vi "Y_XZModefying.vi"() -> ()   [LabVIEW 2013]
uses:
  <vilib>/Instr/_visa.llb/VISA Configure Serial Port (Instr).vi
  <vilib>/Native 3D Graph/xcontrol/3DPC_SurfacePlot.xctl
  <vilib>/Analysis/Matrix/NI_Matrix.lvlib
  <vilib>/Analysis/Matrix/Numeric/Conversions/Array To Matrix - RA.vi
panel:
  in  "Path":path
  out "3D Graph":refnum<class "Base Datatype.lvclass">[](xcontrol)
  in  "ZAdjustStep um":dbl format="%#_13g"
  in  "CurrFluctuationTolerance %":dbl format="%#_13g"
  in  "stop":bool
  in  "ZRoughApproachPerStep um":dbl format="%#_13g"
  in  "ZMovThresholdChange %":dbl format="%#_13g"
  in  "ZApproachingThresholdDecline %":dbl format="%#_13g"
  in  "ZApproachPerStep um":dbl format="%#_13g"
  in  "ZAdjustSpeed um/s":dbl format="%#_13g"
  in  "ConstantCurrPIZ":refnum<visa-resource-name>
  in  "ZApproachSpeed um/s":dbl format="%#_13g"
  in  "YMovSpeed um/s":dbl format="%#_13g"
  in  "XMovSpeed um/s":dbl format="%#_13g"
  in  "Y Length / um":dbl format="%#_13g"
  in  "X Length / um":dbl format="%#_13g"
  in  "Y Resolution":i32
  in  "X Resolution":i32
  in  "Amp":refnum<visa-resource-name>
  in  "Moving":refnum<visa-resource-name>
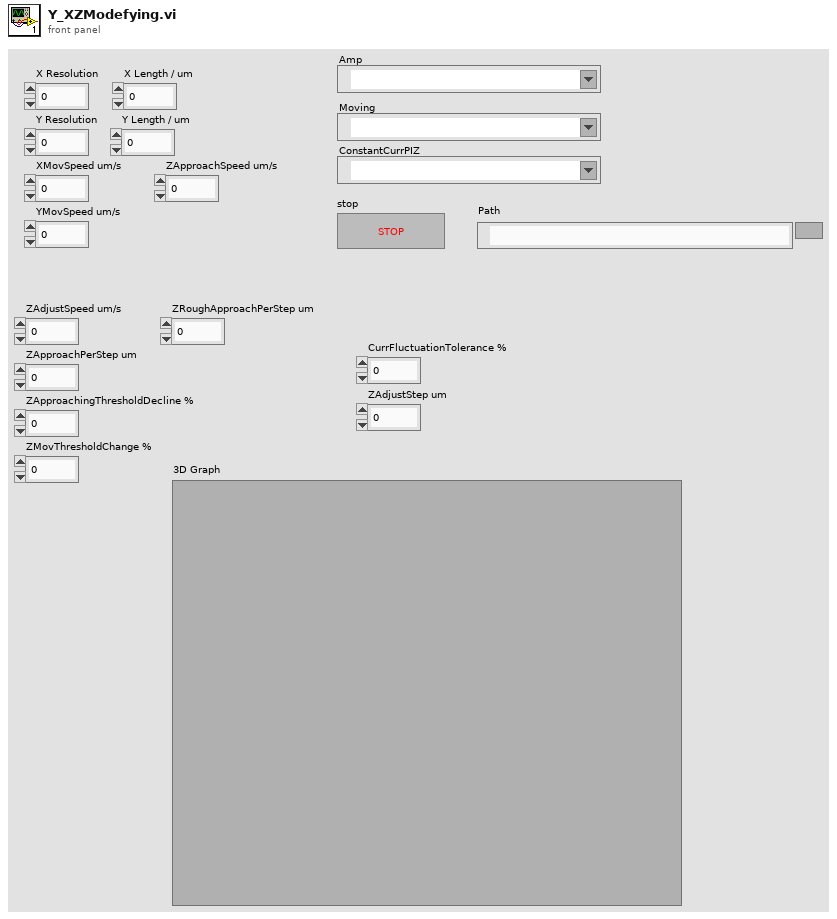
[diagram p1: front panel]
types:
  T1 = enum16{"open", "replace", "create", "open or create", "replace or create", "replace or create with confirmation"}
  T2 = typedef "NI_Matrix.lvlib/RealMatrix.ctl" = dbl[][]
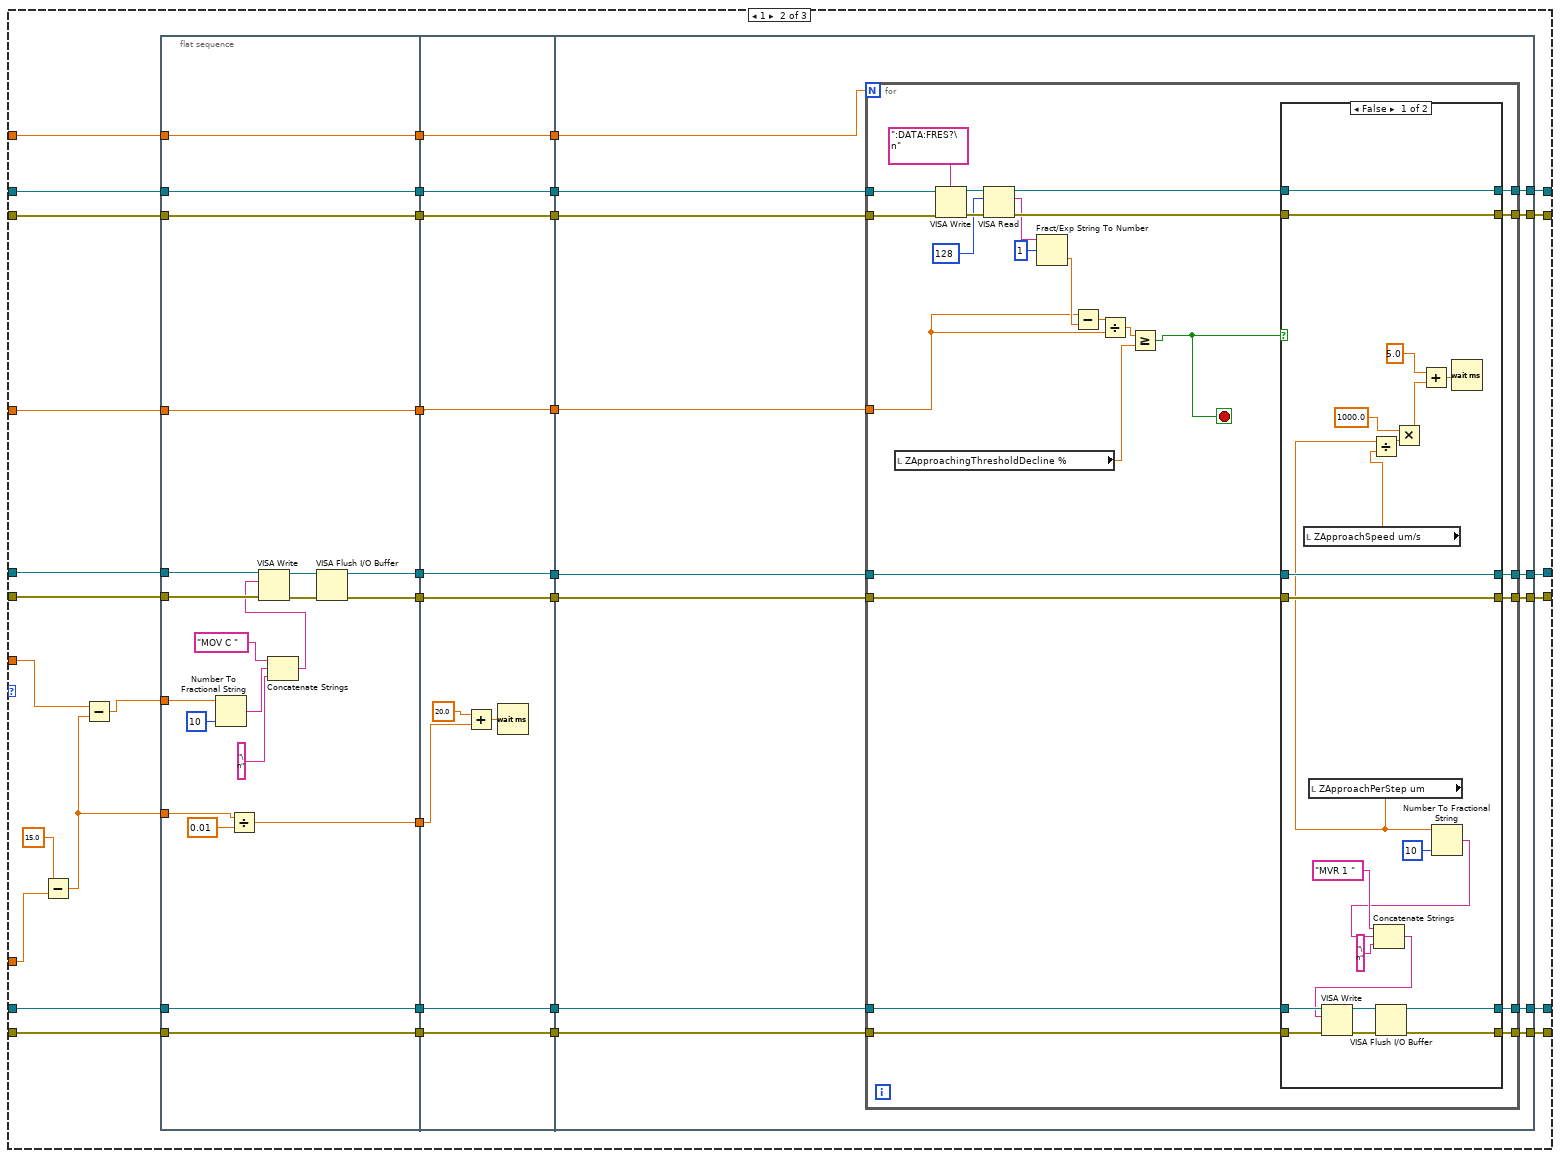
[diagram p5: hidden frame]
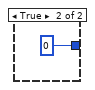
[diagram p9: hidden frame]
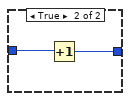
[diagram p10: hidden frame]
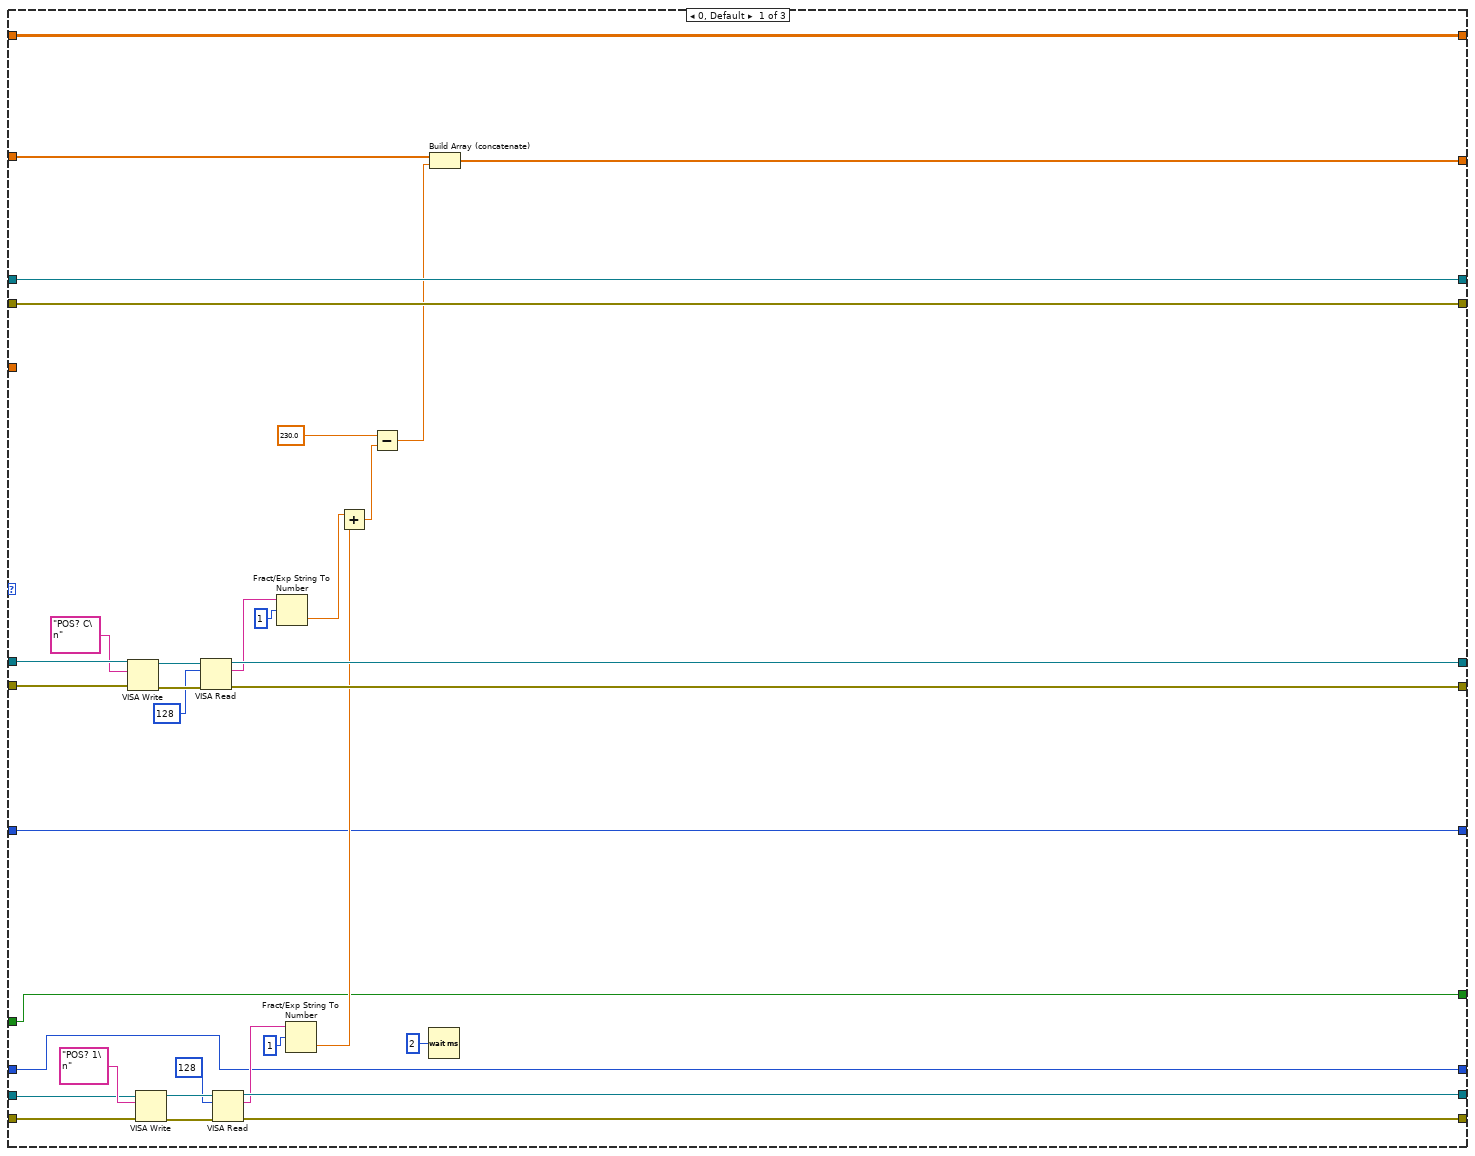
[diagram p11: hidden frame]
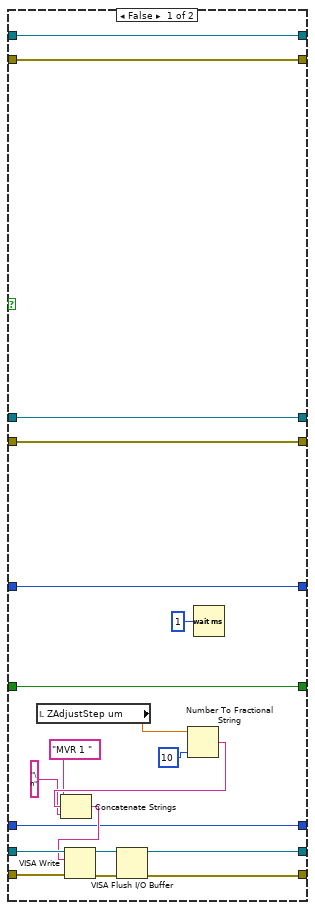
[diagram p12: hidden frame]
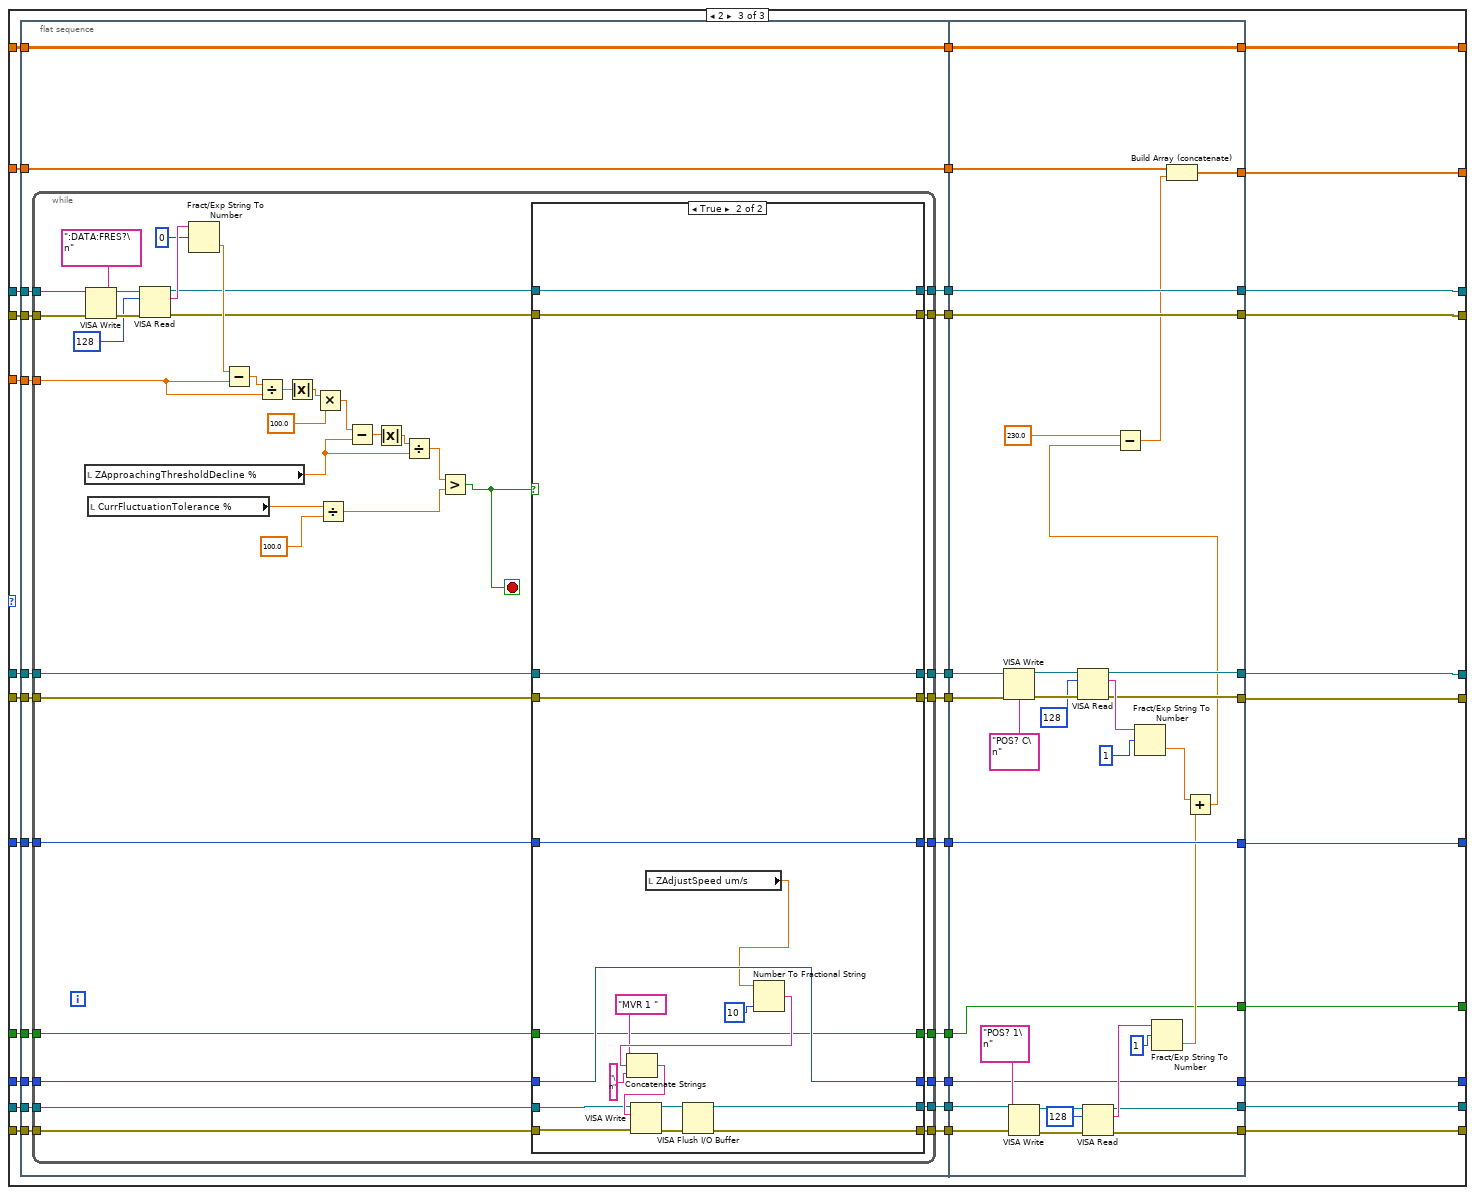
[diagram p13: hidden frame]
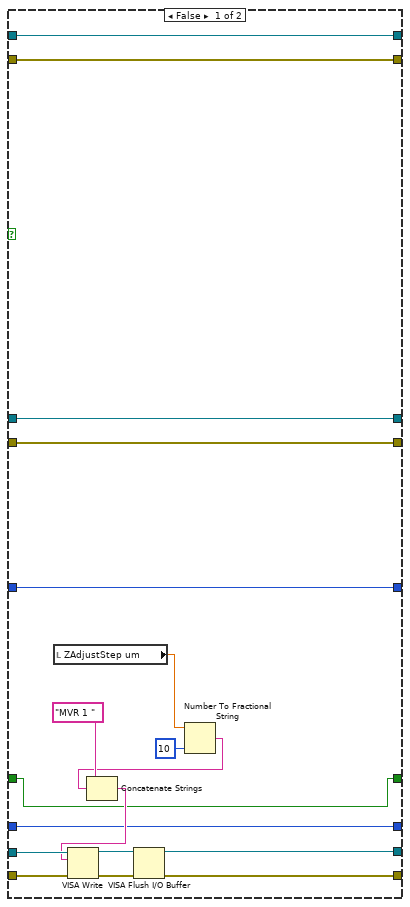
[diagram p14: hidden frame]
diagram:
  n1 = local write "ZApproachingThresholdDecline %"("ZApproachingThresholdDecline %") -> ()
  n2 = local write "ZAdjustStep um"("ZAdjustStep um") -> ()
  n3 = local write "ZMovThresholdChange %"("ZMovThresholdChange %") -> ()
  n4 = local write "X Resolution"("X Resolution") -> ()
  n5 = local write "ZAdjustSpeed um/s"("ZAdjustSpeed um/s") -> ()
  n6 = local write "Y Resolution"("Y Resolution") -> ()
  n7 = local write "ZRoughApproachPerStep um"("ZRoughApproachPerStep um") -> ()
  n8 = local write "ZApproachPerStep um"("ZApproachPerStep um") -> ()
  n9 = call-poly "VISA Configure Serial Port"("VISA resource name"="ConstantCurrPIZ", "baud rate (9600)"=u32 115200) -> ("VISA resource name out"=w12:refnum<visa-resource-name>, "error out"=w11:errorcluster)  [unwired: 12 in]
  n10 = call-poly "VISA Configure Serial Port"("VISA resource name"="Moving", "baud rate (9600)"=u32 115200) -> ("VISA resource name out"=w7:refnum<visa-resource-name>, "error out"=w5:errorcluster)  [unwired: 12 in]
  n11 = call-poly "VISA Configure Serial Port"("VISA resource name"="Amp", "baud rate (9600)"=u32 115200) -> ("VISA resource name out"=w97:refnum<visa-resource-name>, "error out"=w96:errorcluster)  [unwired: 12 in]
  n12 = VISA Write(VISA resource name=w7, write buffer="ERR?\n", error in (no error)=w5) -> (VISA resource name out=w6:refnum<visa-resource-name>, error out=w4:errorcluster)  [unwired: 1 out]
  n13 = VISA Write(VISA resource name=w12, write buffer="ERR?\n", error in (no error)=w11) -> (VISA resource name out=w10:refnum<visa-resource-name>, error out=w9:errorcluster)  [unwired: 1 out]
  n14 = flat-sequence {
    tunnel: w97 -> [w131]
    tunnel: w96 -> [w130]
    tunnel: w6 -> [w101]
    tunnel: w4 -> [w100]
    tunnel: [w129] -> w93
    tunnel: [w128] -> w92
    tunnel: [w127] -> w91
    tunnel: [w126] -> w90
    tunnel: "XMovSpeed um/s" -> [w124]
    tunnel: [w124] -> w88
    tunnel: "YMovSpeed um/s" -> [w123]
    tunnel: [w123] -> w86
    tunnel: w10 -> [w114]
    tunnel: w9 -> [w113]
    tunnel: [w122] -> w83
    tunnel: [w121] -> w82
    tunnel: [w119] -> w81
    tunnel: "ZApproachSpeed um/s" -> [w119]
    tunnel: [w105] -> w56
    tunnel: w93 -> [w134]
    tunnel: w92 -> [w133]
    tunnel: w91 -> [w152]
    tunnel: w90 -> [w151]
    tunnel: [w134] -> w65
    tunnel: [w133] -> w67
    tunnel: [w150] -> w69
    tunnel: [w149] -> w71
    tunnel: w88 -> [_]
    tunnel: w86 -> [_]
    tunnel: w83 -> [w144]
    tunnel: w82 -> [w143]
    tunnel: [w142] -> w73
    tunnel: [w141] -> w75
    tunnel: w81 -> [w135]
    tunnel: w56 -> [w132]
    tunnel: w75 -> [w159]
    tunnel: [w159] -> w74
    tunnel: w73 -> [w158]
    tunnel: [w158] -> w72
    tunnel: w71 -> [w157]
    tunnel: [w157] -> w70
    tunnel: w69 -> [w156]
    tunnel: [w156] -> w68
    tunnel: w67 -> [w155]
    tunnel: [w155] -> w66
    tunnel: w65 -> [w154]
    tunnel: [w154] -> w64
    tunnel: w74 -> [w173]
    tunnel: w72 -> [w174]
    tunnel: w70 -> [w168]
    tunnel: w68 -> [w169]
    tunnel: w66 -> [w175]
    tunnel: w64 -> [w176]
    tunnel: [w167] -> w62
    tunnel: [w166] -> w61
    tunnel: [w165] -> w60
    tunnel: [w164] -> w59
    tunnel: [w163] -> w58
    tunnel: [w162] -> w57
    tunnel: [w161] -> w55
    tunnel: [w160] -> w40
    tunnel: w62 -> [w410]
    tunnel: w61 -> [w409]
    tunnel: w60 -> [w408]
    tunnel: w59 -> [w407]
    tunnel: w58 -> [w406]
    tunnel: w57 -> [w405]
    tunnel: [w370] -> w54
    tunnel: w55 -> [w370]
    tunnel: [w385] -> w51
    tunnel: [w384] -> w49
    tunnel: [w383] -> w47
    tunnel: [w382] -> w45
    tunnel: [w381] -> w43
    tunnel: [w380] -> w41
    tunnel: w40 -> [w371]
    tunnel: w54 -> [w759]
    tunnel: [w759] -> w53
    tunnel: [w758] -> w52
    tunnel: w51 -> [w758]
    tunnel: [w757] -> w50
    tunnel: w49 -> [w757]
    tunnel: [w756] -> w48
    tunnel: w47 -> [w756]
    tunnel: [w755] -> w46
    tunnel: w45 -> [w755]
    tunnel: [w754] -> w44
    tunnel: w43 -> [w754]
    tunnel: [w753] -> w42
    tunnel: w41 -> [w753]
    tunnel: [dbl[][] []] -> w37
    tunnel: [dbl[] []] -> w36
    tunnel: [w745] -> w2
    tunnel: [w744] -> w1
    tunnel: w53 -> [w781]
    tunnel: w52 -> [w783]
    tunnel: w50 -> [w782]
    tunnel: w48 -> [w787]
    tunnel: w46 -> [w786]
    tunnel: w44 -> [w785]
    tunnel: w42 -> [w784]
    tunnel: w37 -> [w779]
    tunnel: w36 -> [w780]
    tunnel: [w778] -> w34
    tunnel: [w777] -> w33
    tunnel: [w769] -> w32
    tunnel: [w771] -> w31
    tunnel: [w776] -> w30
    tunnel: [w775] -> w29
    tunnel: [w774] -> w22
    tunnel: [w773] -> w21
    tunnel: w2 -> [w764]
    tunnel: w1 -> [w763]
    tunnel: w34 -> [w1424]
    tunnel: w33 -> [w1423]
    tunnel: w32 -> [w1413]
    tunnel: w31 -> [w1412]
    tunnel: w30 -> [w1421]
    tunnel: w29 -> [w1420]
    tunnel: [w1417] -> w28
    tunnel: [w1416] -> w27
    tunnel: [w1415] -> w26
    tunnel: [w1414] -> w25
    tunnel: [w1413] -> w24
    tunnel: [w1412] -> w23
    tunnel: w22 -> [w1411]
    tunnel: w21 -> [w1410]
    tunnel: [w1408] -> w20
    tunnel: [w1407] -> w19
    tunnel: w28 -> [w1436]
    tunnel: w27 -> [w1435]
    tunnel: w26 -> [w1430]
    tunnel: w25 -> [w1429]
    tunnel: [w1432] -> w16
    tunnel: [w1431] -> w15
    tunnel: [w1430] -> w14
    tunnel: [w1429] -> w13
    tunnel: [w1428] -> _
    tunnel: w24 -> [w1428]
    tunnel: [w1427] -> _
    tunnel: w23 -> [w1427]
    tunnel: w20 -> [w1426]
    tunnel: w19 -> [w1425]
    tunnel: [w1426] -> w18
    tunnel: [w1425] -> w17
    frame #0 {
      n15 = VISA Write(VISA resource name=w114, write buffer="POS?\n", error in (no error)=w113) -> (VISA resource name out=w117:refnum<visa-resource-name>, error out=w116:errorcluster)  [unwired: 1 out]
      n16 = VISA Read(VISA resource name=w117, byte count=u32 128, error in (no error)=w116) -> (VISA resource name out=w112:refnum<visa-resource-name>, read buffer=w109:string, error out=w111:errorcluster)  [unwired: 1 out]
      n17 = Fract/Exp String To Number(string=w109, offset=1) -> (number=w107:dbl)  [unwired: 2 in, 1 out]
      n18 = Divide(x=w107, y=0.005) -> (x/y=w102:dbl)
      n19 = Wait (ms)(milliseconds to wait=u32 4000) -> ()  [unwired: 1 out]
      n20 = VISA Write(VISA resource name=w101, write buffer="SVO A 1 B 1 C 1\nMOV A 0\nMOV B 0\nMOV C 0\n", error in (no error)=w100) -> (VISA resource name out=w129:refnum<visa-resource-name>, error out=w128:errorcluster)  [unwired: 1 out]
      n21 = Add(x=w102, y=100.0) -> (x+y=w105:dbl)
      n22 = VISA Write(VISA resource name=w112, write buffer="SVO 1 1\nMOV 1 0\n", error in (no error)=w111) -> (VISA resource name out=w122:refnum<visa-resource-name>, error out=w121:errorcluster)  [unwired: 1 out]
      n23 = VISA Write(VISA resource name=w131, write buffer=":SENS:FUNC 'VOLT'\n:SENS:VOLT:RANG 20\n:FORM:ELEM READ\n\n:SENS:CURR:NPLC 0.01\n:CALC:STAT OFF\n:SYSTEM:LSYN:STAT OFF\n\n:DISP:ENAB 1\n:SYST:ZCH OFF\n:INIT:CONT ON\n", error in (no error)=w130) -> (VISA resource name out=w127:refnum<visa-resource-name>, error out=w126:errorcluster)  [unwired: 1 out]
    }
    frame #1 {
      n24 = VISA Write(VISA resource name=w152, write buffer=":DATA:FRES?\n", error in (no error)=w151) -> (VISA resource name out=w148:refnum<visa-resource-name>, error out=w147:errorcluster)  [unwired: 1 out]
      n25 = Number To Fractional String(number=w135, precision (6)=i16 10) -> (F-format string=w137:string)  [unwired: 2 in]
      n26 = Concatenate Strings("VEL 1 ", w137, "\n" ("string")) -> (w136:string)
      n27 = Wait (ms)(milliseconds to wait=w132) -> ()  [unwired: 1 out]
      n28 = VISA Read(VISA resource name=w148, byte count=u32 128, error in (no error)=w147) -> (VISA resource name out=w150:refnum<visa-resource-name>, error out=w149:errorcluster)  [unwired: 2 out]
      n29 = VISA Write(VISA resource name=w144, write buffer=w136, error in (no error)=w143) -> (VISA resource name out=w142:refnum<visa-resource-name>, error out=w141:errorcluster)  [unwired: 1 out]
    }
    frame #2 {
      n30 = Wait (ms)(milliseconds to wait=u32 10) -> ()  [unwired: 1 out]
    }
    frame #3 {
      n31 = local read "ZApproachPerStep um"() -> (w170:dbl)
      n32 = Divide(x=30.0, y=w170) -> (x/y=w171:dbl)
      n33 = Round Toward -Infinity(1:w171) -> (0:w160:dbl)
      n34 = while {
        tunnel: w176 -> [w192]
        tunnel: w175 -> [w190]
        tunnel: w169 -> [w197]
        tunnel: w168 -> [w196]
        tunnel: w174 -> [w199]
        tunnel: w173 -> [w198]
        tunnel: w160 -> [w201]
        tunnel: w170 -> [w200]
        tunnel: [w183] -> w165
        tunnel: [w182] -> w164
        tunnel: [w181] -> w167
        tunnel: [w180] -> w166
        tunnel: [w179] -> w163
        tunnel: [w178] -> w162
        tunnel: [w177] -> w161
        stop <- w186 stop-if-true
        n35 = for {
          N: 50 -> [_]
          tunnel: w197 -> [w206]
          tunnel: w196 -> [w205]
          tunnel: [w204] -> w194
          tunnel: [w203] -> w193
          tunnel: [w202] -> w177
          # "Reference Curr"
          n36 = VISA Write(VISA resource name=w206, write buffer=":DATA:FRES?\n", error in (no error)=w205) -> (VISA resource name out=w211:refnum<visa-resource-name>, error out=w210:errorcluster)  [unwired: 1 out]
          n37 = VISA Read(VISA resource name=w211, byte count=u32 128, error in (no error)=w210) -> (VISA resource name out=w204:refnum<visa-resource-name>, read buffer=w207:string, error out=w203:errorcluster)  [unwired: 1 out]
          n38 = Fract/Exp String To Number(string=w207) -> (number=w202:dbl)  [unwired: 3 in, 1 out]
        }
        n39 = for {
          N: w201 -> [_]
          tunnel: w200 -> [_]
          tunnel: w199 -> [w320]
          tunnel: w198 -> [w319]
          tunnel: w177 -> [w331]
          tunnel: w194 -> [w336]
          tunnel: w193 -> [w335]
          tunnel: [w326] -> w185
          tunnel: [w325] -> w184
          tunnel: w192 -> [w324]
          tunnel: [w323] -> w191
          tunnel: w190 -> [w322]
          tunnel: [w321] -> w189
          tunnel: [w317] -> w188
          tunnel: [w316] -> w187
          tunnel: [w315] -> w186
          stop <- w315 stop-if-true
          n40 = local read "ZApproachingThresholdDecline %"() -> (w329:dbl)
          n41 = local read "ZApproachPerStep um"() -> (w318:dbl)
          n42 = VISA Write(VISA resource name=w336, write buffer=":DATA:FRES?\n", error in (no error)=w335) -> (VISA resource name out=w340:refnum<visa-resource-name>, error out=w339:errorcluster)  [unwired: 1 out]
          n43 = VISA Read(VISA resource name=w340, byte count=u32 128, error in (no error)=w339) -> (VISA resource name out=w328:refnum<visa-resource-name>, read buffer=w337:string, error out=w327:errorcluster)  [unwired: 1 out]
          n44 = Fract/Exp String To Number(string=w337) -> (number=w334:dbl)  [unwired: 3 in, 1 out]
          n45 = Subtract(x=w334, y=w331) -> (x-y=w333:dbl)
          n46 = Absolute Value(x=w333) -> (abs(x)=w332:dbl)
          n47 = Divide(x=w332, y=w331) -> (x/y=w330:dbl)
          n48 = Greater Or Equal?(x=w330, y=w329) -> (x >= y?=w315:bool)
          n49 = case shown="False" w315 {
            tunnel: w328 -> [w363 w369]
            tunnel: w327 -> [w362 w368]
            tunnel: [w363 w369] -> w326
            tunnel: [w362 w368] -> w325
            tunnel: w324 -> [w361 w367]
            tunnel: [w361 w367] -> w323
            tunnel: w322 -> [w360 w366]
            tunnel: [w360 w366] -> w321
            tunnel: w320 -> [w359 w365]
            tunnel: w319 -> [w358 w364]
            tunnel: w318 -> [w344 _]
            tunnel: [w352 w365] -> w317
            tunnel: [w351 w364] -> w316
            frame False {
              n50 = local read "ZApproachSpeed um/s"() -> (w343:dbl)
              n51 = Number To Fractional String(number=w344, precision (6)=i16 10) -> (F-format string=w356:string)  [unwired: 2 in]
              n52 = Divide(x=w343, y=w344) -> (x/y=w346:dbl)
              n53 = Concatenate Strings("MVR 1 ", w356, "\n") -> (w353:string)
              n54 = Multiply(x=w346, y=1000.0) -> (x*y=w342:dbl)
              n55 = VISA Write(VISA resource name=w359, write buffer=w353, error in (no error)=w358) -> (VISA resource name out=w350:refnum<visa-resource-name>, error out=w349:errorcluster)  [unwired: 1 out]
              n56 = Add(x=5.0, y=w342) -> (x+y=w348:dbl)
              n57 = VISA Flush I/O Buffer(VISA resource name=w350, error in (no error)=w349) -> (VISA resource name out=w352:refnum<visa-resource-name>, error out=w351:errorcluster)  [unwired: 1 in]
              n58 = Wait (ms)(milliseconds to wait=w348) -> ()  [unwired: 1 out]
            }
            frame True {
            }
          }
        }
        n59 = case shown="False" w186 {
          tunnel: w191 -> [w239 w314]
          tunnel: w189 -> [w238 w313]
          tunnel: w188 -> [w237 w310]
          tunnel: w187 -> [w236 w309]
          tunnel: w185 -> [w243 w312]
          tunnel: w184 -> [w241 w311]
          tunnel: [w216 w314] -> w183
          tunnel: [w215 w313] -> w182
          tunnel: [w242 w312] -> w181
          tunnel: [w240 w311] -> w180
          tunnel: [w214 w310] -> w179
          tunnel: [w213 w309] -> w178
          frame False {
            n60 = flat-sequence {
              tunnel: [w265] -> w229
              tunnel: [w264] -> w227
              tunnel: [w263] -> w225
              tunnel: [w262] -> w223
              tunnel: [w257] -> w221
              tunnel: [w256] -> w219
              tunnel: w236 -> [w254]
              tunnel: w237 -> [w253]
              tunnel: w238 -> [w262]
              tunnel: w239 -> [w263]
              tunnel: w241 -> [w264]
              tunnel: w243 -> [w265]
              tunnel: [w244] -> w217
              tunnel: w229 -> [w276]
              tunnel: [w276] -> w228
              tunnel: w227 -> [w275]
              tunnel: [w275] -> w226
              tunnel: w225 -> [w274]
              tunnel: [w274] -> w224
              tunnel: w223 -> [w273]
              tunnel: [w273] -> w222
              tunnel: w221 -> [w272]
              tunnel: [w272] -> w220
              tunnel: w219 -> [w271]
              tunnel: [w271] -> w218
              tunnel: w217 -> [w266]
              tunnel: w228 -> [w297]
              tunnel: w226 -> [w296]
              tunnel: w224 -> [w282]
              tunnel: w222 -> [w281]
              tunnel: w220 -> [w295]
              tunnel: w218 -> [w294]
              tunnel: [w297] -> w235
              tunnel: [w296] -> w234
              tunnel: [w286] -> w233
              tunnel: [w285] -> w232
              tunnel: [w279] -> w231
              tunnel: [w278] -> w230
              tunnel: [w277] -> w212
              tunnel: [w307] -> w240
              tunnel: [w308] -> w242
              tunnel: w235 -> [w308]
              tunnel: w234 -> [w307]
              tunnel: w233 -> [w304]
              tunnel: w232 -> [w303]
              tunnel: w231 -> [w306]
              tunnel: w230 -> [w305]
              tunnel: [w306] -> w216
              tunnel: [w305] -> w215
              tunnel: [w304] -> w214
              tunnel: [w303] -> w213
              tunnel: w212 -> [w301]
              frame #0 {
                n61 = VISA Write(VISA resource name=w253, write buffer="VEL 1 10\nPOS?\n", error in (no error)=w254) -> (VISA resource name out=w251:refnum<visa-resource-name>, error out=w250:errorcluster)  [unwired: 1 out]
                n62 = VISA Flush I/O Buffer(VISA resource name=w251, error in (no error)=w250) -> (VISA resource name out=w249:refnum<visa-resource-name>, error out=w248:errorcluster)  [unwired: 1 in]
                n63 = VISA Read(VISA resource name=w249, byte count=u32 128, error in (no error)=w248) -> (VISA resource name out=w259:refnum<visa-resource-name>, read buffer=w246:string, error out=w258:errorcluster)  [unwired: 1 out]
                n64 = Fract/Exp String To Number(string=w246, offset=1) -> (number=w244:dbl)  [unwired: 2 in, 1 out]
                n65 = VISA Write(VISA resource name=w259, write buffer="MOV 1 0\n", error in (no error)=w258) -> (VISA resource name out=w261:refnum<visa-resource-name>, error out=w260:errorcluster)  [unwired: 1 out]
                n66 = VISA Flush I/O Buffer(VISA resource name=w261, error in (no error)=w260) -> (VISA resource name out=w257:refnum<visa-resource-name>, error out=w256:errorcluster)  [unwired: 1 in]
              }
              frame #1 {
                n67 = Divide(x=w266, y=0.01) -> (x/y=w269:dbl)
                n68 = Add(x=w269, y=10.0) -> (x+y=w267:dbl)
                n69 = Wait (ms)(milliseconds to wait=w267) -> ()  [unwired: 1 out]
              }
              frame #2 {
                n70 = local read "ZApproachSpeed um/s"() -> (w277:dbl)
                n71 = VISA Write(VISA resource name=w282, write buffer="MVR C 25\n", error in (no error)=w281) -> (VISA resource name out=w284:refnum<visa-resource-name>, error out=w283:errorcluster)  [unwired: 1 out]
                n72 = VISA Flush I/O Buffer(VISA resource name=w284, error in (no error)=w283) -> (VISA resource name out=w279:refnum<visa-resource-name>, error out=w278:errorcluster)  [unwired: 1 in]
                n73 = Number To Fractional String(number=w277, precision (6)=i16 10) -> (F-format string=w288:string)  [unwired: 2 in]
                n74 = Concatenate Strings("VEL 1 " ("write buffer"), w288, "\n" ("string")) -> (w290:string)
                n75 = VISA Write(VISA resource name=w295, write buffer=w290, error in (no error)=w294) -> (VISA resource name out=w293:refnum<visa-resource-name>, error out=w292:errorcluster)  [unwired: 1 out]
                n76 = VISA Flush I/O Buffer(VISA resource name=w293, error in (no error)=w292) -> (VISA resource name out=w286:refnum<visa-resource-name>, error out=w285:errorcluster)  [unwired: 1 in]
              }
              frame #3 {
                n77 = Divide(x=0.025, y=w301) -> (x/y=w300:dbl)
                n78 = Add(x=w300, y=10.0) -> (x+y=w298:dbl)
                n79 = Wait (ms)(milliseconds to wait=w298) -> ()  [unwired: 1 out]
              }
            }
          }
          frame True {
          }
        }
      }
    }
    frame #4 {
      n80 = VISA Write(VISA resource name=w408, write buffer="POS? C\n", error in (no error)=w407) -> (VISA resource name out=w402:refnum<visa-resource-name>, error out=w401:errorcluster)  [unwired: 1 out]
      n81 = VISA Write(VISA resource name=w406, write buffer="POS?\n", error in (no error)=w405) -> (VISA resource name out=w400:refnum<visa-resource-name>, error out=w399:errorcluster)  [unwired: 1 out]
      n82 = VISA Read(VISA resource name=w400, byte count=u32 128, error in (no error)=w399) -> (VISA resource name out=w392:refnum<visa-resource-name>, read buffer=w396:string, error out=w391:errorcluster)  [unwired: 1 out]
      n83 = VISA Read(VISA resource name=w402, byte count=u32 128, error in (no error)=w401) -> (VISA resource name out=w394:refnum<visa-resource-name>, read buffer=w379:string, error out=w393:errorcluster)  [unwired: 1 out]
      n84 = Fract/Exp String To Number(string=w379, offset=1) -> (number=w377:dbl)  [unwired: 2 in, 1 out]
      n85 = Fract/Exp String To Number(string=w396, offset=1) -> (number=w372:dbl)  [unwired: 2 in, 1 out]
      n86 = Less?(x=w372, y=10.0) -> (x < y?=w376:bool)
      n87 = Greater?(x=w372, y=20.0) -> (0:w375:bool)
      n88 = Boolean To (0,1)(Boolean=w376) -> (0, 1=w387:i16)
      n89 = Boolean To (0,1)(Boolean=w375) -> (0, 1=w390:i16)
      n90 = Multiply(x=w390, y=i16 2) -> (x*y=w386:i16)
      n91 = Add(x=w387, y=w386) -> (x+y=w388:i16)
      n92 = case shown="2" w388 {
        tunnel: w410 -> [w416 w443 w590]
        tunnel: w409 -> [w415 w441 w587]
        tunnel: w372 -> [_ w452 w602]
        tunnel: w394 -> [w414 w451 w606]
        tunnel: w393 -> [w413 w450 w605]
        tunnel: w392 -> [w412 w440 w604]
        tunnel: w391 -> [w411 w439 w603]
        tunnel: [w416 w422 w558] -> w385
        tunnel: [w415 w421 w557] -> w384
        tunnel: [w414 w420 w556] -> w383
        tunnel: [w413 w419 w555] -> w382
        tunnel: [w412 w418 w554] -> w381
        tunnel: [w411 w417 w553] -> w380
        tunnel: w377 -> [_ w449 w584]
        tunnel: w371 -> [_ w426 w576]
        tunnel: w370 -> [_ w425 w568]
        frame 0, Default {
        }
        frame 1 {
          n93 = Subtract(x=15.0, y=w452) -> (x-y=w436:dbl)
          n94 = Subtract(x=w449, y=w436) -> (x-y=w448:dbl)
          n95 = flat-sequence {
            tunnel: w451 -> [w473]
            tunnel: w450 -> [w472]
            tunnel: w448 -> [w469]
            tunnel: [w463] -> w447
            tunnel: [w462] -> w446
            tunnel: [w461] -> w444
            tunnel: w443 -> [w461]
            tunnel: [w460] -> w442
            tunnel: w441 -> [w460]
            tunnel: w440 -> [w459]
            tunnel: w439 -> [w458]
            tunnel: [w459] -> w438
            tunnel: [w458] -> w437
            tunnel: w436 -> [w457]
            tunnel: [w455] -> w435
            tunnel: [w454] -> w427
            tunnel: w426 -> [w454]
            tunnel: w425 -> [w453]
            tunnel: [w453] -> w423
            tunnel: w447 -> [w481]
            tunnel: w446 -> [w480]
            tunnel: w444 -> [w477]
            tunnel: w442 -> [w476]
            tunnel: w438 -> [w479]
            tunnel: w437 -> [w478]
            tunnel: w435 -> [w483]
            tunnel: [w481] -> w434
            tunnel: [w480] -> w433
            tunnel: [w479] -> w432
            tunnel: [w478] -> w431
            tunnel: [w477] -> w430
            tunnel: [w476] -> w429
            tunnel: [w475] -> w428
            tunnel: w427 -> [w475]
            tunnel: [w474] -> w424
            tunnel: w423 -> [w474]
            tunnel: w429 -> [w492]
            tunnel: w430 -> [w493]
            tunnel: w431 -> [w496]
            tunnel: w432 -> [w497]
            tunnel: w433 -> [w494]
            tunnel: w434 -> [w495]
            tunnel: w428 -> [w498]
            tunnel: w424 -> [w491]
            tunnel: [w490] -> w422
            tunnel: [w489] -> w421
            tunnel: [w488] -> w420
            tunnel: [w487] -> w419
            tunnel: [w486] -> w418
            tunnel: [w485] -> w417
            frame #0 {
              n96 = Number To Fractional String(number=w469, precision (6)=i16 10) -> (F-format string=w470:string)  [unwired: 2 in]
              n97 = Divide(x=w457, y=0.01) -> (x/y=w455:dbl)
              n98 = Concatenate Strings("MOV C ", w470, "\n" ("string")) -> (w466:string)
              n99 = VISA Write(VISA resource name=w473, write buffer=w466, error in (no error)=w472) -> (VISA resource name out=w464:refnum<visa-resource-name>, error out=w465:errorcluster)  [unwired: 1 out]
              n100 = VISA Flush I/O Buffer(VISA resource name=w464, error in (no error)=w465) -> (VISA resource name out=w463:refnum<visa-resource-name>, error out=w462:errorcluster)  [unwired: 1 in]
            }
            frame #1 {
              n101 = Add(x=20.0, y=w483) -> (x+y=w484:dbl)
              n102 = Wait (ms)(milliseconds to wait=w484) -> ()  [unwired: 1 out]
            }
            frame #2 {
              n103 = for {
                N: w498 -> [_]
                tunnel: w497 -> [w502]
                tunnel: w496 -> [w501]
                tunnel: w495 -> [w509]
                tunnel: w494 -> [w508]
                tunnel: w493 -> [w524]
                tunnel: w492 -> [w523]
                tunnel: w491 -> [w512]
                tunnel: [w506] -> w490
                tunnel: [w505] -> w489
                tunnel: [w504] -> w488
                tunnel: [w503] -> w487
                tunnel: [w500] -> w486
                tunnel: [w499] -> w485
                stop <- w507 stop-if-true
                n104 = local read "ZApproachingThresholdDecline %"() -> (w510:dbl)
                n105 = VISA Write(VISA resource name=w524, write buffer=":DATA:FRES?\n", error in (no error)=w523) -> (VISA resource name out=w521:refnum<visa-resource-name>, error out=w520:errorcluster)  [unwired: 1 out]
                n106 = VISA Read(VISA resource name=w521, byte count=u32 128, error in (no error)=w520) -> (VISA resource name out=w518:refnum<visa-resource-name>, read buffer=w516:string, error out=w517:errorcluster)  [unwired: 1 out]
                n107 = Fract/Exp String To Number(string=w516, offset=1) -> (number=w514:dbl)  [unwired: 2 in, 1 out]
                n108 = Subtract(x=w512, y=w514) -> (x-y=w513:dbl)
                n109 = Divide(x=w513, y=w512) -> (x/y=w511:dbl)
                n110 = Greater Or Equal?(x=w511, y=w510) -> (x >= y?=w507:bool)
                n111 = case shown="False" w507 {
                  tunnel: w518 -> [w546 w552]
                  tunnel: w517 -> [w545 w551]
                  tunnel: w509 -> [w544 w550]
                  tunnel: w508 -> [w543 w549]
                  tunnel: [w546 w552] -> w506
                  tunnel: [w545 w551] -> w505
                  tunnel: [w544 w550] -> w504
                  tunnel: [w543 w549] -> w503
                  tunnel: w502 -> [w542 w548]
                  tunnel: w501 -> [w541 w547]
                  tunnel: [w533 w548] -> w500
                  tunnel: [w532 w547] -> w499
                  frame False {
                    n112 = local read "ZApproachSpeed um/s"() -> (w531:dbl)
                    n113 = local read "ZApproachPerStep um"() -> (w530:dbl)
                    n114 = Divide(x=w530, y=w531) -> (x/y=w527:dbl)
                    n115 = Multiply(x=1000.0, y=w527) -> (x*y=w525:dbl)
                    n116 = Add(x=5.0, y=w525) -> (x+y=w529:dbl)
                    n117 = Number To Fractional String(number=w530, precision (6)=i16 10) -> (F-format string=w538:string)  [unwired: 2 in]
                    n118 = Concatenate Strings("MVR 1 ", w538, "\n" ("string")) -> (w536:string)
                    n119 = VISA Write(VISA resource name=w542, write buffer=w536, error in (no error)=w541) -> (VISA resource name out=w535:refnum<visa-resource-name>, error out=w534:errorcluster)  [unwired: 1 out]
                    n120 = VISA Flush I/O Buffer(VISA resource name=w535, error in (no error)=w534) -> (VISA resource name out=w533:refnum<visa-resource-name>, error out=w532:errorcluster)  [unwired: 1 in]
                    n121 = Wait (ms)(milliseconds to wait=w529) -> ()  [unwired: 1 out]
                  }
                  frame True {
                  }
                }
              }
            }
          }
        }
        frame 2 {
          n122 = flat-sequence {
            tunnel: w606 -> [w617]
            tunnel: w605 -> [w616]
            tunnel: w604 -> [w629]
            tunnel: w603 -> [w628]
            tunnel: w602 -> [w612]
            tunnel: [w624] -> w601
            tunnel: [w623] -> w600
            tunnel: [w618] -> w599
            tunnel: [w617] -> w595
            tunnel: [w616] -> w593
            tunnel: [w615] -> w591
            tunnel: w590 -> [w615]
            tunnel: [w614] -> w588
            tunnel: w587 -> [w614]
            tunnel: w584 -> [w610]
            tunnel: [w613] -> w583
            tunnel: [w609] -> w581
            tunnel: [w608] -> w577
            tunnel: w576 -> [w608]
            tunnel: [w607] -> w569
            tunnel: w568 -> [w607]
            tunnel: w601 -> [w640]
            tunnel: w600 -> [w639]
            tunnel: w599 -> [w642]
            tunnel: [w640] -> w598
            tunnel: [w639] -> w597
            tunnel: [w638] -> w596
            tunnel: w595 -> [w638]
            tunnel: [w637] -> w594
            tunnel: w593 -> [w637]
            tunnel: [w636] -> w592
            tunnel: w591 -> [w636]
            tunnel: [w635] -> w589
            tunnel: w588 -> [w635]
            tunnel: w583 -> [w634]
            tunnel: [w634] -> w582
            tunnel: w581 -> [w633]
            tunnel: [w633] -> w580
            tunnel: [w632] -> w578
            tunnel: w577 -> [w632]
            tunnel: w569 -> [w631]
            tunnel: [w631] -> w566
            tunnel: w598 -> [w645]
            tunnel: w597 -> [w644]
            tunnel: w596 -> [w664]
            tunnel: w594 -> [w663]
            tunnel: w592 -> [w648]
            tunnel: w589 -> [w647]
            tunnel: [w658] -> w586
            tunnel: [w657] -> w585
            tunnel: w582 -> [w656]
            tunnel: w580 -> [w652]
            tunnel: [w650] -> w579
            tunnel: w578 -> [w649]
            tunnel: [w649] -> w575
            tunnel: [w648] -> w572
            tunnel: [w647] -> w570
            tunnel: [w646] -> w567
            tunnel: w566 -> [w646]
            tunnel: [w645] -> w562
            tunnel: [w644] -> w561
            tunnel: w586 -> [w668]
            tunnel: w585 -> [w667]
            tunnel: w579 -> [w673]
            tunnel: w575 -> [w672]
            tunnel: [w672] -> w574
            tunnel: [w671] -> w573
            tunnel: w572 -> [w671]
            tunnel: [w670] -> w571
            tunnel: w570 -> [w670]
            tunnel: w567 -> [w669]
            tunnel: [w669] -> w565
            tunnel: [w668] -> w564
            tunnel: [w667] -> w563
            tunnel: w562 -> [w666]
            tunnel: w561 -> [w665]
            tunnel: [w666] -> w560
            tunnel: [w665] -> w559
            tunnel: w574 -> [w689]
            tunnel: w573 -> [w688]
            tunnel: w571 -> [w687]
            tunnel: w565 -> [w686]
            tunnel: w564 -> [w685]
            tunnel: w563 -> [w684]
            tunnel: w560 -> [w683]
            tunnel: w559 -> [w682]
            tunnel: [w681] -> w558
            tunnel: [w680] -> w557
            tunnel: [w679] -> w556
            tunnel: [w678] -> w555
            tunnel: [w677] -> w554
            tunnel: [w676] -> w553
            frame #0 {
              n123 = local read "ZApproachSpeed um/s"() -> (w621:dbl)
              n124 = Subtract(x=w612, y=15.0) -> (x-y=w622:dbl)
              n125 = VISA Write(VISA resource name=w629, write buffer="MOV 1 15\n", error in (no error)=w628) -> (VISA resource name out=w625:refnum<visa-resource-name>, error out=w626:errorcluster)  [unwired: 1 out]
              n126 = VISA Flush I/O Buffer(VISA resource name=w625, error in (no error)=w626) -> (VISA resource name out=w624:refnum<visa-resource-name>, error out=w623:errorcluster)  [unwired: 1 in]
              n127 = Subtract(x=w612, y=2.0) -> (x-y=w609:dbl)
              n128 = Divide(x=w622, y=w621) -> (x/y=w620:dbl)
              n129 = Add(x=w610, y=w609) -> (x+y=w613:dbl)
              n130 = Multiply(x=w620, y=1000.0) -> (x*y=w618:dbl)
            }
            frame #1 {
              n131 = Add(x=w642, y=10.0) -> (x+y=w643:dbl)
              n132 = Wait (ms)(milliseconds to wait=w643) -> ()  [unwired: 1 out]
            }
            frame #2 {
              n133 = Divide(x=w652, y=0.01) -> (x/y=w650:dbl)
              n134 = Number To Fractional String(number=w656, precision (6)=i16 10) -> (F-format string=w654:string)  [unwired: 2 in]
              n135 = Concatenate Strings("MOV C " ("string"), w654, "\n" ("string")) -> (w660:string)
              n136 = VISA Write(VISA resource name=w664, write buffer=w660, error in (no error)=w663) -> (VISA resource name out=w662:refnum<visa-resource-name>, error out=w661:errorcluster)  [unwired: 1 out]
              n137 = VISA Flush I/O Buffer(VISA resource name=w662, error in (no error)=w661) -> (VISA resource name out=w658:refnum<visa-resource-name>, error out=w657:errorcluster)  [unwired: 1 in]
            }
            frame #3 {
              n138 = Add(x=w673, y=10.0) -> (x+y=w674:dbl)
              n139 = Wait (ms)(milliseconds to wait=w674) -> ()  [unwired: 1 out]
            }
            frame #4 {
              n140 = for {
                N: w689 -> [_]
                tunnel: w688 -> [w709]
                tunnel: w687 -> [w708]
                tunnel: w686 -> [w705]
                tunnel: w685 -> [w699]
                tunnel: w684 -> [w698]
                tunnel: w683 -> [w697]
                tunnel: w682 -> [w696]
                tunnel: [w695] -> w681
                tunnel: [w694] -> w680
                tunnel: [w693] -> w679
                tunnel: [w692] -> w678
                tunnel: [w691] -> w677
                tunnel: [w690] -> w676
                stop <- w702 stop-if-true
                n141 = local read "ZApproachingThresholdDecline %"() -> (w703:dbl)
                n142 = VISA Write(VISA resource name=w709, write buffer=":DATA:FRES?\n", error in (no error)=w708) -> (VISA resource name out=w714:refnum<visa-resource-name>, error out=w713:errorcluster)  [unwired: 1 out]
                n143 = VISA Read(VISA resource name=w714, byte count=u32 128, error in (no error)=w713) -> (VISA resource name out=w701:refnum<visa-resource-name>, read buffer=w711:string, error out=w700:errorcluster)  [unwired: 1 out]
                n144 = Fract/Exp String To Number(string=w711, offset=0) -> (number=w707:dbl)  [unwired: 2 in, 1 out]
                n145 = Subtract(x=w705, y=w707) -> (x-y=w706:dbl)
                n146 = Divide(x=w706, y=w705) -> (x/y=w704:dbl)
                n147 = Greater Or Equal?(x=w704, y=w703) -> (x >= y?=w702:bool)
                n148 = case shown="False" w702 {
                  tunnel: w701 -> [w737 w743]
                  tunnel: w700 -> [w736 w742]
                  tunnel: w699 -> [w735 w741]
                  tunnel: w698 -> [w734 w740]
                  tunnel: w697 -> [w731 w739]
                  tunnel: w696 -> [w730 w738]
                  tunnel: [w737 w743] -> w695
                  tunnel: [w736 w742] -> w694
                  tunnel: [w735 w741] -> w693
                  tunnel: [w734 w740] -> w692
                  tunnel: [w729 w739] -> w691
                  tunnel: [w728 w738] -> w690
                  frame False {
                    n149 = local read "ZApproachPerStep um"() -> (w722:dbl)
                    n150 = local read "ZApproachSpeed um/s"() -> (w721:dbl)
                    n151 = Divide(x=w722, y=w721) -> (x/y=w720:dbl)
                    n152 = Multiply(x=w720, y=1000.0) -> (x*y=w717:dbl)
                    n153 = Number To Fractional String(number=w722, precision (6)=i16 10) -> (F-format string=w725:string)  [unwired: 2 in]
                    n154 = Concatenate Strings("MVR 1 ", w725, "\n" ("string")) -> (w723:string)
                    n155 = VISA Write(VISA resource name=w731, write buffer=w723, error in (no error)=w730) -> (VISA resource name out=w733:refnum<visa-resource-name>, error out=w732:errorcluster)  [unwired: 1 out]
                    n156 = VISA Flush I/O Buffer(VISA resource name=w733, error in (no error)=w732) -> (VISA resource name out=w729:refnum<visa-resource-name>, error out=w728:errorcluster)  [unwired: 1 in]
                    n157 = Add(x=w717, y=5.0) -> (x+y=w718:dbl)
                    n158 = Wait (ms)(milliseconds to wait=w718) -> ()  [unwired: 1 out]
                  }
                  frame True {
                  }
                }
              }
            }
          }
        }
      }
    }
    frame #5 {
      n159 = Wait (ms)(milliseconds to wait=u32 20) -> ()  [unwired: 1 out]
      n160 = call <vilib>:"Check if File or Folder Exists.vi"("path"="Path") -> ("file or folder exists?"=w749:bool)  [unwired: 8 in, 2 out]
      n161 = case shown="False" w749 {
        tunnel: "Path" -> [w761 w762]
        tunnel: [w760 w762] -> w747
        frame False {
          n162 = Delete(path (use dialog)=w761) -> (deleted path=w760:path)  [unwired: 4 in, 2 out]
        }
        frame True {
        }
      }
      n163 = Open/Create/Replace File(file path (use dialog)=w747, operation (0:open)=T1."create") -> (refnum out=w745:refnum<file>, error out=w744:errorcluster)  [unwired: 4 in, 1 out]
    }
    frame #6 {
      n164 = while {
        tunnel: w787 -> [w828]
        tunnel: w786 -> [w826]
        tunnel: w785 -> [w832]
        tunnel: w784 -> [w831]
        tunnel: w783 -> [w824]
        tunnel: w782 -> [w822]
        tunnel: w781 -> [w814]
        shift-right: [w804] -> w769
        shift-left: w779 -> [w803]
        shift-right: [w802] -> w771
        shift-left: w780 -> [w808]
        tunnel: [w798] -> w774
        tunnel: [w797] -> w773
        tunnel: [w796] -> w776
        tunnel: [w795] -> w775
        tunnel: [w794] -> w778
        tunnel: [w793] -> w777
        tunnel: w764 -> [w790]
        tunnel: w763 -> [w788]
        i -> [w835]
        stop <- w839 stop-if-true
        n165 = local read "Y Resolution"() -> (w836:i32)
        n166 = flat-sequence {
          tunnel: [w850] -> w837
          tunnel: w836 -> [w844]
          tunnel: w835 -> [w847]
          tunnel: [w859] -> w834
          tunnel: [w858] -> w833
          tunnel: w832 -> [w858]
          tunnel: w831 -> [w857]
          tunnel: [w857] -> w830
          tunnel: [w856] -> w829
          tunnel: w828 -> [w856]
          tunnel: [w855] -> w827
          tunnel: w826 -> [w855]
          tunnel: [w854] -> w825
          tunnel: w824 -> [w854]
          tunnel: [w853] -> w823
          tunnel: w822 -> [w853]
          tunnel: [w852] -> w815
          tunnel: w814 -> [w852]
          tunnel: w803 -> [w851]
          tunnel: [w851] -> w812
          tunnel: [w844] -> w811
          tunnel: [w849] -> w810
          tunnel: w808 -> [w843]
          tunnel: [w843] -> w807
          tunnel: [w842] -> w800
          tunnel: [w841] -> w791
          tunnel: w790 -> [w841]
          tunnel: [w840] -> w789
          tunnel: w788 -> [w840]
          tunnel: w834 -> [w868]
          tunnel: w833 -> [w876]
          tunnel: w830 -> [w875]
          tunnel: w829 -> [w887]
          tunnel: w827 -> [w886]
          tunnel: w825 -> [w874]
          tunnel: w823 -> [w873]
          tunnel: [w878] -> w817
          tunnel: [w877] -> w816
          tunnel: [w876] -> w821
          tunnel: [w875] -> w820
          tunnel: [w874] -> w819
          tunnel: [w873] -> w818
          tunnel: [w872] -> w813
          tunnel: w815 -> [w872]
          tunnel: [w871] -> w805
          tunnel: w812 -> [w871]
          tunnel: [w869] -> w801
          tunnel: [w870] -> w792
          tunnel: w811 -> [w870]
          tunnel: w810 -> [w869]
          tunnel: [w868] -> w809
          tunnel: w807 -> [w867]
          tunnel: [w867] -> w806
          tunnel: [w866] -> w799
          tunnel: w800 -> [w866]
          tunnel: [w865] -> _
          tunnel: w791 -> [w865]
          tunnel: w789 -> [w864]
          tunnel: [w864] -> _
          frame #0 {
            n167 = local read "Y Length / um"() -> (w861:dbl)
            n168 = Greater Or Equal?(x=w847, y=w844) -> (x >= y?=w850:bool)
            n169 = Quotient & Remainder(x=w847, y=2) -> (x-y*floor(x/y)=w846:i32)  [unwired: 1 out]
            n170 = Equal?(x=w846, y=0) -> (x = y?=w842:bool)
            n171 = case shown="False" w842 {
              tunnel: [w862 0] -> w849
              tunnel: w844 -> [w862 _]
              frame False {
              }
              frame True {
              }
            }
            n172 = Divide(x=w861, y=w847) -> (x/y=w860:dbl)
            n173 = Multiply(x=w860, y=w844) -> (x*y=w859:dbl)
          }
          frame #1 {
            n174 = Number To Fractional String(number=w868, precision (6)=i16 10) -> (F-format string=w884:string)  [unwired: 2 in]
            n175 = Concatenate Strings("MOV B " ("string"), w884, "\n" ("string")) -> (w881:string)
            n176 = VISA Write(VISA resource name=w887, write buffer=w881, error in (no error)=w886) -> (VISA resource name out=w880:refnum<visa-resource-name>, error out=w879:errorcluster)  [unwired: 1 out]
            n177 = VISA Flush I/O Buffer(VISA resource name=w880, error in (no error)=w879) -> (VISA resource name out=w878:refnum<visa-resource-name>, error out=w877:errorcluster)  [unwired: 1 in]
          }
        }
        n178 = while {
          tunnel: ["stop"] -> w838
          tunnel: w821 -> [w943]
          tunnel: w820 -> [w942]
          tunnel: w819 -> [w941]
          tunnel: w818 -> [w940]
          tunnel: w817 -> [w945]
          tunnel: w816 -> [w944]
          tunnel: w813 -> [w931]
          tunnel: w809 -> [w912]
          tunnel: [w907] -> w797
          tunnel: [w906] -> w798
          tunnel: [w904] -> w796
          tunnel: [w903] -> w795
          shift-right: [w902] -> w802
          shift-left: w806 -> [w910]
          shift-right: [w905] -> w804
          shift-left: w805 -> [w901]
          tunnel: [w900] -> w794
          tunnel: [w899] -> w793
          shift-right: [w890] -> _
          shift-left: w801 -> [w898]
          tunnel: w799 -> [w895]
          tunnel: [w889] -> _
          tunnel: w792 -> [w888]
          stop <- w949 stop-if-true
          n179 = local read "X Resolution"() -> (w920:i32)
          n180 = local read "X Length / um"() -> (w947:dbl)
          n181 = Greater Or Equal?(x=w898, y=w920) -> (x >= y?=w919:bool)
          n182 = Less?(x=w898, y=0) -> (x < y?=w917:bool)
          n183 = Divide(x=w947, y=w920) -> (x/y=w946:dbl)
          n184 = Or(x=w919, y=w917) -> (x .or. y?=w918:bool)
          n185 = flat-sequence {
            tunnel: w946 -> [w958]
            tunnel: w945 -> [w978]
            tunnel: w944 -> [w977]
            tunnel: w943 -> [w965]
            tunnel: w942 -> [w964]
            tunnel: w941 -> [w962]
            tunnel: w940 -> [w961]
            tunnel: [w974] -> w939
            tunnel: [w973] -> w938
            tunnel: w898 -> [w966]
            tunnel: [w965] -> w935
            tunnel: [w964] -> w934
            tunnel: w931 -> [w963]
            tunnel: [w963] -> w930
            tunnel: [w962] -> w928
            tunnel: [w961] -> w927
            tunnel: w901 -> [w960]
            tunnel: [w960] -> w924
            tunnel: w898 -> [w959]
            tunnel: [w959] -> w922
            tunnel: w888 -> [w955]
            tunnel: [w958] -> w914
            tunnel: [w957] -> w913
            tunnel: w912 -> [w957]
            tunnel: w910 -> [w956]
            tunnel: [w956] -> w909
            tunnel: [w955] -> w897
            tunnel: w895 -> [w954]
            tunnel: [w954] -> w893
            tunnel: w939 -> [w993]
            tunnel: w938 -> [w992]
            tunnel: [w993] -> w937
            tunnel: [w992] -> w936
            tunnel: w935 -> [w990]
            tunnel: w934 -> [w989]
            tunnel: [w990] -> w933
            tunnel: [w989] -> w932
            tunnel: w930 -> [w988]
            tunnel: [w988] -> w929
            tunnel: w928 -> [w987]
            tunnel: w927 -> [w986]
            tunnel: [w987] -> w926
            tunnel: [w986] -> w925
            tunnel: w924 -> [w985]
            tunnel: [w985] -> w923
            tunnel: w922 -> [w984]
            tunnel: [w984] -> w921
            tunnel: [w983] -> w915
            tunnel: w914 -> [w983]
            tunnel: w913 -> [w982]
            tunnel: [w982] -> w911
            tunnel: w909 -> [w981]
            tunnel: [w981] -> w908
            tunnel: w897 -> [w980]
            tunnel: [w980] -> w896
            tunnel: [w979] -> w894
            tunnel: w893 -> [w979]
            tunnel: w937 -> [w1028]
            tunnel: w936 -> [w1027]
            tunnel: w933 -> [w1019]
            tunnel: w932 -> [w1018]
            tunnel: w929 -> [w1010]
            tunnel: w926 -> [w1048]
            tunnel: w925 -> [w1047]
            tunnel: w923 -> [w1013]
            tunnel: w921 -> [w1017]
            tunnel: w915 -> [w1015]
            tunnel: w911 -> [w1016]
            tunnel: w908 -> [w1011]
            tunnel: [w1006] -> w905
            tunnel: [w1005] -> w902
            tunnel: [w1004] -> w906
            tunnel: [w1003] -> w907
            tunnel: [w1002] -> w904
            tunnel: [w1001] -> w903
            tunnel: [w1000] -> w900
            tunnel: [w999] -> w899
            tunnel: [w998] -> w891
            tunnel: w896 -> [w997]
            tunnel: [w996] -> w889
            tunnel: w894 -> [w995]
            tunnel: [w994] -> w892
            frame #0 {
              n186 = Multiply(x=w958, y=w966) -> (x*y=w967:dbl)
              n187 = Number To Fractional String(number=w967, precision (6)=i16 10) -> (F-format string=w970:string)  [unwired: 2 in]
              n188 = Concatenate Strings("MOV A " ("string"), w970, "\n" ("string")) -> (w972:string)
              n189 = VISA Write(VISA resource name=w978, write buffer=w972, error in (no error)=w977) -> (VISA resource name out=w976:refnum<visa-resource-name>, error out=w975:errorcluster)  [unwired: 1 out]
              n190 = VISA Flush I/O Buffer(VISA resource name=w976, error in (no error)=w975) -> (VISA resource name out=w974:refnum<visa-resource-name>, error out=w973:errorcluster)  [unwired: 1 in]
            }
            frame #1 {
              n191 = Wait (ms)(milliseconds to wait=u32 1) -> ()  [unwired: 1 out]
            }
            frame #2 {
              n192 = local read "ZMovThresholdChange %"() -> (w1033:dbl)
              n193 = VISA Write(VISA resource name=w1048, write buffer=":DATA:FRES?\n", error in (no error)=w1047) -> (VISA resource name out=w1045:refnum<visa-resource-name>, error out=w1044:errorcluster)  [unwired: 1 out]
              n194 = VISA Read(VISA resource name=w1045, byte count=u32 128, error in (no error)=w1044) -> (VISA resource name out=w1042:refnum<visa-resource-name>, read buffer=w1040:string, error out=w1041:errorcluster)  [unwired: 1 out]
              n195 = Build Array(w1015, w1016) -> (w1014:dbl[])
              n196 = Fract/Exp String To Number(string=w1040, offset=0) -> (number=w1038:dbl)  [unwired: 2 in, 1 out]
              n197 = Subtract(x=w1010, y=w1038) -> (x-y=w1037:dbl)
              n198 = Divide(x=w1037, y=w1010) -> (x/y=w1036:dbl)
              n199 = Multiply(x=w1036, y=100.0) -> (x*y=w1034:dbl)
              n200 = Divide(x=w1034, y=w1033) -> (x/y=w1032:dbl)
              n201 = Build Array (concatenate)(w1013, w1014) -> (w1012:dbl[][])
              n202 = local write "CurrFluctuationTolerance %"("CurrFluctuationTolerance %") -> ()
              n203 = Subtract(x=w1032, y=1.0) -> (x-y=w1030:dbl)
              n204 = Divide(x="CurrFluctuationTolerance %", y=100.0) -> (x/y=w1009:dbl)
              n205 = Negate(x=w1009) -> (-x=w1029:dbl)
              n206 = Greater?(x=w1030, y=w1009) -> (0:w1026:bool)
              n207 = Less?(x=w1030, y=w1029) -> (x < y?=w1024:bool)
              n208 = Boolean To (0,1)(Boolean=w1026) -> (0, 1=w1025:i16)
              n209 = Boolean To (0,1)(Boolean=w1024) -> (0, 1=w1023:i16)
              n210 = Multiply(x=w1023, y=i16 2) -> (x*y=w1021:i16)
              n211 = Add(x=w1025, y=w1021) -> (x+y=w1020:i16)
              n212 = case shown="1" w1020 {
                tunnel: w1042 -> [w1062 w1108 w1274]
                tunnel: w1041 -> [w1061 w1107 w1273]
                tunnel: w1028 -> [w1080 w1110 w1271]
                tunnel: w1027 -> [w1079 w1109 w1270]
                tunnel: w1019 -> [w1074 w1112 w1268]
                tunnel: w1018 -> [w1073 w1111 w1267]
                tunnel: w1017 -> [w1051 w1091 w1269]
                tunnel: w1012 -> [w1052 w1116 w1266]
                tunnel: w1011 -> [w1056 w1113 w1265]
                tunnel: [w1072 w1093 w1252] -> w1000
                tunnel: [w1071 w1092 w1250] -> w999
                tunnel: [w1070 w1095 w1256] -> w1002
                tunnel: [w1069 w1094 w1253] -> w1001
                tunnel: [w1062 w1103 w1260] -> w1004
                tunnel: [w1061 w1100 w1258] -> w1003
                tunnel: [w1053 w1104 w1262] -> w1005
                tunnel: w1010 -> [_ w1106 w1272]
                tunnel: [w1052 w1105 w1261] -> w1006
                tunnel: [w1051 w1089 w1247] -> w998
                tunnel: w997 -> [w1050 w1088 w1246]
                tunnel: [w1050 w1086 w1244] -> w996
                tunnel: w995 -> [w1049 w1085 w1243]
                tunnel: [w1049 w1083 w1241] -> w994
                frame 0, Default {
                  n213 = VISA Write(VISA resource name=w1080, write buffer="POS? C\n", error in (no error)=w1079) -> (VISA resource name out=w1082:refnum<visa-resource-name>, error out=w1081:errorcluster)  [unwired: 1 out]
                  n214 = VISA Write(VISA resource name=w1074, write buffer="POS? 1\n", error in (no error)=w1073) -> (VISA resource name out=w1077:refnum<visa-resource-name>, error out=w1076:errorcluster)  [unwired: 1 out]
                  n215 = VISA Read(VISA resource name=w1082, byte count=u32 128, error in (no error)=w1081) -> (VISA resource name out=w1070:refnum<visa-resource-name>, read buffer=w1063:string, error out=w1069:errorcluster)  [unwired: 1 out]
                  n216 = VISA Read(VISA resource name=w1077, byte count=u32 128, error in (no error)=w1076) -> (VISA resource name out=w1072:refnum<visa-resource-name>, read buffer=w1065:string, error out=w1071:errorcluster)  [unwired: 1 out]
                  n217 = Fract/Exp String To Number(string=w1063, offset=1) -> (number=w1058:dbl)  [unwired: 2 in, 1 out]
                  n218 = Fract/Exp String To Number(string=w1065, offset=1) -> (number=w1057:dbl)  [unwired: 2 in, 1 out]
                  n219 = Add(x=w1058, y=w1057) -> (x+y=w1059:dbl)
                  n220 = Subtract(x=230.0, y=w1059) -> (x-y=w1055:dbl)
                  n221 = Wait (ms)(milliseconds to wait=u32 2) -> ()  [unwired: 1 out]
                  n222 = Build Array (concatenate)(w1056, w1055) -> (w1053:dbl[])
                }
                frame 1 {
                  n223 = flat-sequence {
                    tunnel: w1116 -> [w1137]
                    tunnel: [w1137] -> w1115
                    tunnel: [w1136] -> w1114
                    tunnel: w1113 -> [w1136]
                    tunnel: w1112 -> [w1135]
                    tunnel: w1111 -> [w1134]
                    tunnel: w1110 -> [w1133]
                    tunnel: w1109 -> [w1132]
                    tunnel: w1108 -> [w1131]
                    tunnel: w1107 -> [w1130]
                    tunnel: w1106 -> [w1129]
                    tunnel: [w1128] -> w1102
                    tunnel: [w1127] -> w1101
                    tunnel: [w1126] -> w1099
                    tunnel: [w1125] -> w1098
                    tunnel: [w1124] -> w1097
                    tunnel: [w1123] -> w1096
                    tunnel: w1091 -> [w1122]
                    tunnel: [w1121] -> w1090
                    tunnel: w1088 -> [w1120]
                    tunnel: [w1119] -> w1087
                    tunnel: w1085 -> [w1118]
                    tunnel: [w1117] -> w1084
                    tunnel: w1115 -> [w1240]
                    tunnel: w1114 -> [w1239]
                    tunnel: [w1240] -> w1105
                    tunnel: [w1238] -> w1104
                    tunnel: [w1237] -> w1103
                    tunnel: w1102 -> [w1237]
                    tunnel: [w1236] -> w1100
                    tunnel: w1101 -> [w1236]
                    tunnel: w1099 -> [w1229]
                    tunnel: w1098 -> [w1228]
                    tunnel: w1097 -> [w1235]
                    tunnel: w1096 -> [w1234]
                    tunnel: [w1225] -> w1095
                    tunnel: [w1224] -> w1094
                    tunnel: [w1218] -> w1093
                    tunnel: [w1217] -> w1092
                    tunnel: [w1210] -> w1089
                    tunnel: w1090 -> [w1210]
                    tunnel: w1087 -> [w1209]
                    tunnel: [w1209] -> w1086
                    tunnel: w1084 -> [w1208]
                    tunnel: [w1208] -> w1083
                    frame #0 {
                      n224 = while {
                        tunnel: w1135 -> [w1166]
                        tunnel: w1134 -> [w1165]
                        tunnel: w1133 -> [w1168]
                        tunnel: w1132 -> [w1167]
                        tunnel: w1131 -> [w1172]
                        tunnel: w1130 -> [w1171]
                        tunnel: w1129 -> [w1162]
                        tunnel: [w1149] -> w1128
                        tunnel: [w1148] -> w1127
                        tunnel: [w1147] -> w1126
                        tunnel: [w1146] -> w1125
                        tunnel: [w1145] -> w1124
                        tunnel: [w1144] -> w1123
                        tunnel: w1122 -> [w1143]
                        tunnel: [w1142] -> w1121
                        tunnel: w1120 -> [w1141]
                        tunnel: [w1140] -> w1119
                        tunnel: w1118 -> [w1139]
                        tunnel: [w1138] -> w1117
                        stop <- w1150 stop-if-true
                        n225 = local read "ZApproachingThresholdDecline %"() -> (w1153:dbl)
                        n226 = VISA Write(VISA resource name=w1172, write buffer=":DATA:FRES?\n", error in (no error)=w1171) -> (VISA resource name out=w1177:refnum<visa-resource-name>, error out=w1176:errorcluster)  [unwired: 1 out]
                        n227 = local read "CurrFluctuationTolerance %"() -> (w1157:dbl)
                        n228 = VISA Read(VISA resource name=w1177, byte count=u32 128, error in (no error)=w1176) -> (VISA resource name out=w1170:refnum<visa-resource-name>, read buffer=w1174:string, error out=w1169:errorcluster)  [unwired: 1 out]
                        n229 = Fract/Exp String To Number(string=w1174, offset=0) -> (number=w1164:dbl)  [unwired: 2 in, 1 out]
                        n230 = Subtract(x=w1164, y=w1162) -> (x-y=w1163:dbl)
                        n231 = Divide(x=w1163, y=w1162) -> (x/y=w1161:dbl)
                        n232 = Absolute Value(x=w1161) -> (abs(x)=w1160:dbl)
                        n233 = Divide(x=w1157, y=100.0) -> (x/y=w1151:dbl)
                        n234 = Multiply(x=w1160, y=100.0) -> (x*y=w1158:dbl)
                        n235 = Subtract(x=w1158, y=w1153) -> (x-y=w1155:dbl)
                        n236 = Absolute Value(x=w1155) -> (abs(x)=w1154:dbl)
                        n237 = Divide(x=w1154, y=w1153) -> (x/y=w1152:dbl)
                        n238 = Greater?(x=w1152, y=w1151) -> (0:w1150:bool)
                        n239 = case shown="True" w1150 {
                          tunnel: w1170 -> [w1198 w1207]
                          tunnel: w1169 -> [w1197 w1206]
                          tunnel: w1168 -> [w1196 w1205]
                          tunnel: w1167 -> [w1195 w1204]
                          tunnel: w1166 -> [w1194 w1203]
                          tunnel: w1165 -> [w1193 w1202]
                          tunnel: [w1198 w1207] -> w1149
                          tunnel: [w1197 w1206] -> w1148
                          tunnel: [w1196 w1205] -> w1147
                          tunnel: [w1195 w1204] -> w1146
                          tunnel: [w1190 w1203] -> w1145
                          tunnel: [w1189 w1202] -> w1144
                          tunnel: w1143 -> [w1181 w1201]
                          tunnel: [w1181 w1201] -> w1142
                          tunnel: w1141 -> [w1180 w1199]
                          tunnel: [w1180 w1199] -> w1140
                          tunnel: [w1179 w1200] -> w1138
                          tunnel: w1139 -> [w1179 w1200]
                          frame False {
                            n240 = local read "ZAdjustStep um"() -> (w1187:dbl)
                            n241 = Number To Fractional String(number=w1187, precision (6)=i16 10) -> (F-format string=w1185:string)  [unwired: 2 in]
                            n242 = Concatenate Strings("MVR 1 " ("string"), w1185, "\n" ("string")) -> (w1188:string)
                            n243 = VISA Write(VISA resource name=w1194, write buffer=w1188, error in (no error)=w1193) -> (VISA resource name out=w1192:refnum<visa-resource-name>, error out=w1191:errorcluster)  [unwired: 1 out]
                            n244 = VISA Flush I/O Buffer(VISA resource name=w1192, error in (no error)=w1191) -> (VISA resource name out=w1190:refnum<visa-resource-name>, error out=w1189:errorcluster)  [unwired: 1 in]
                            n245 = Wait (ms)(milliseconds to wait=u32 1) -> ()  [unwired: 1 out]
                          }
                          frame True {
                          }
                        }
                      }
                    }
                    frame #1 {
                      n246 = VISA Write(VISA resource name=w1229, write buffer="POS? C\n", error in (no error)=w1228) -> (VISA resource name out=w1231:refnum<visa-resource-name>, error out=w1230:errorcluster)  [unwired: 1 out]
                      n247 = VISA Write(VISA resource name=w1235, write buffer="POS? 1\n", error in (no error)=w1234) -> (VISA resource name out=w1233:refnum<visa-resource-name>, error out=w1232:errorcluster)  [unwired: 1 out]
                      n248 = VISA Read(VISA resource name=w1231, byte count=u32 128, error in (no error)=w1230) -> (VISA resource name out=w1225:refnum<visa-resource-name>, read buffer=w1223:string, error out=w1224:errorcluster)  [unwired: 1 out]
                      n249 = VISA Read(VISA resource name=w1233, byte count=u32 128, error in (no error)=w1232) -> (VISA resource name out=w1218:refnum<visa-resource-name>, read buffer=w1216:string, error out=w1217:errorcluster)  [unwired: 1 out]
                      n250 = Fract/Exp String To Number(string=w1223, offset=1) -> (number=w1214:dbl)  [unwired: 2 in, 1 out]
                      n251 = Fract/Exp String To Number(string=w1216, offset=1) -> (number=w1213:dbl)  [unwired: 2 in, 1 out]
                      n252 = Add(x=w1214, y=w1213) -> (x+y=w1212:dbl)
                      n253 = Subtract(x=230.0, y=w1212) -> (x-y=w1211:dbl)
                      n254 = Build Array (concatenate)(w1239, w1211) -> (w1238:dbl[])
                    }
                  }
                }
                frame 2 {
                  n255 = flat-sequence {
                    tunnel: w1274 -> [w1295]
                    tunnel: w1273 -> [w1294]
                    tunnel: w1272 -> [w1293]
                    tunnel: w1271 -> [w1292]
                    tunnel: w1270 -> [w1291]
                    tunnel: w1269 -> [w1290]
                    tunnel: w1268 -> [w1289]
                    tunnel: w1267 -> [w1288]
                    tunnel: w1266 -> [w1287]
                    tunnel: w1265 -> [w1286]
                    tunnel: [w1287] -> w1264
                    tunnel: [w1286] -> w1263
                    tunnel: [w1285] -> w1259
                    tunnel: [w1284] -> w1257
                    tunnel: [w1283] -> w1255
                    tunnel: [w1282] -> w1254
                    tunnel: [w1281] -> w1251
                    tunnel: [w1280] -> w1249
                    tunnel: [w1279] -> w1248
                    tunnel: w1246 -> [w1278]
                    tunnel: [w1277] -> w1245
                    tunnel: w1243 -> [w1276]
                    tunnel: [w1275] -> w1242
                    tunnel: w1264 -> [w1404]
                    tunnel: w1263 -> [w1406]
                    tunnel: [w1405] -> w1262
                    tunnel: [w1404] -> w1261
                    tunnel: [w1403] -> w1260
                    tunnel: w1259 -> [w1403]
                    tunnel: [w1402] -> w1258
                    tunnel: w1257 -> [w1402]
                    tunnel: [w1387] -> w1256
                    tunnel: w1255 -> [w1389]
                    tunnel: [w1386] -> w1253
                    tunnel: w1254 -> [w1388]
                    tunnel: [w1383] -> w1252
                    tunnel: w1251 -> [w1385]
                    tunnel: [w1382] -> w1250
                    tunnel: w1249 -> [w1384]
                    tunnel: w1248 -> [w1381]
                    tunnel: [w1381] -> w1247
                    tunnel: w1245 -> [w1375]
                    tunnel: [w1375] -> w1244
                    tunnel: w1242 -> [w1374]
                    tunnel: [w1374] -> w1241
                    frame #0 {
                      n256 = while {
                        tunnel: w1295 -> [w1330]
                        tunnel: w1294 -> [w1329]
                        tunnel: w1293 -> [w1323]
                        tunnel: w1292 -> [w1311]
                        tunnel: w1291 -> [w1310]
                        tunnel: w1290 -> [w1309]
                        tunnel: w1289 -> [w1308]
                        tunnel: w1288 -> [w1307]
                        tunnel: [w1306] -> w1281
                        tunnel: [w1305] -> w1280
                        tunnel: [w1304] -> w1283
                        tunnel: [w1303] -> w1282
                        tunnel: [w1302] -> w1285
                        tunnel: [w1301] -> w1284
                        tunnel: [w1300] -> w1279
                        tunnel: w1278 -> [w1299]
                        tunnel: [w1298] -> w1277
                        tunnel: w1276 -> [w1297]
                        tunnel: [w1296] -> w1275
                        stop <- w1314 stop-if-true
                        n257 = local read "ZApproachingThresholdDecline %"() -> (w1319:dbl)
                        n258 = VISA Write(VISA resource name=w1330, write buffer=":DATA:FRES?\n", error in (no error)=w1329) -> (VISA resource name out=w1335:refnum<visa-resource-name>, error out=w1334:errorcluster)  [unwired: 1 out]
                        n259 = local read "CurrFluctuationTolerance %"() -> (w1315:dbl)
                        n260 = VISA Read(VISA resource name=w1335, byte count=u32 128, error in (no error)=w1334) -> (VISA resource name out=w1313:refnum<visa-resource-name>, read buffer=w1332:string, error out=w1312:errorcluster)  [unwired: 1 out]
                        n261 = Fract/Exp String To Number(string=w1332, offset=0) -> (number=w1324:dbl)  [unwired: 2 in, 1 out]
                        n262 = Subtract(x=w1324, y=w1323) -> (x-y=w1328:dbl)
                        n263 = Divide(x=w1328, y=w1323) -> (x/y=w1327:dbl)
                        n264 = Absolute Value(x=w1327) -> (abs(x)=w1326:dbl)
                        n265 = Multiply(x=w1326, y=100.0) -> (x*y=w1320:dbl)
                        n266 = Divide(x=w1315, y=100.0) -> (x/y=w1318:dbl)
                        n267 = Subtract(x=w1320, y=w1319) -> (x-y=w1322:dbl)
                        n268 = Absolute Value(x=w1322) -> (abs(x)=w1321:dbl)
                        n269 = Divide(x=w1321, y=w1319) -> (x/y=w1317:dbl)
                        n270 = Greater?(x=w1317, y=w1318) -> (0:w1314:bool)
                        n271 = case shown="True" w1314 {
                          tunnel: w1313 -> [w1354 w1360]
                          tunnel: w1312 -> [w1353 w1359]
                          tunnel: w1311 -> [w1352 w1362]
                          tunnel: w1310 -> [w1351 w1361]
                          tunnel: w1309 -> [w1350 w1358]
                          tunnel: w1308 -> [w1349 w1366]
                          tunnel: w1307 -> [w1348 w1365]
                          tunnel: [w1345 w1364] -> w1306
                          tunnel: [w1344 w1363] -> w1305
                          tunnel: [w1352 w1362] -> w1304
                          tunnel: [w1351 w1361] -> w1303
                          tunnel: [w1354 w1360] -> w1302
                          tunnel: [w1353 w1359] -> w1301
                          tunnel: [w1350 w1358] -> w1300
                          tunnel: w1299 -> [w1338 w1357]
                          tunnel: [w1338 w1357] -> w1298
                          tunnel: w1297 -> [w1337 w1356]
                          tunnel: [w1337 w1356] -> w1296
                          frame False {
                            n272 = local read "ZAdjustStep um"() -> (w1340:dbl)
                            n273 = Number To Fractional String(number=w1340, precision (6)=i16 10) -> (F-format string=w1341:string)  [unwired: 2 in]
                            n274 = Concatenate Strings("MVR 1 " ("string"), w1341) -> (w1343:string)  [unwired: 1 in]
                            n275 = VISA Write(VISA resource name=w1349, write buffer=w1343, error in (no error)=w1348) -> (VISA resource name out=w1347:refnum<visa-resource-name>, error out=w1346:errorcluster)  [unwired: 1 out]
                            n276 = VISA Flush I/O Buffer(VISA resource name=w1347, error in (no error)=w1346) -> (VISA resource name out=w1345:refnum<visa-resource-name>, error out=w1344:errorcluster)  [unwired: 1 in]
                          }
                          frame True {
                            n277 = local read "ZAdjustSpeed um/s"() -> (w1355:dbl)
                            n278 = Number To Fractional String(number=w1355, precision (6)=i16 10) -> (F-format string=w1369:string)  [unwired: 2 in]
                            n279 = Concatenate Strings("MVR 1 " ("string"), w1369, "\n" ("string")) -> (w1371:string)
                            n280 = VISA Write(VISA resource name=w1366, write buffer=w1371, error in (no error)=w1365) -> (VISA resource name out=w1373:refnum<visa-resource-name>, error out=w1372:errorcluster)  [unwired: 1 out]
                            n281 = VISA Flush I/O Buffer(VISA resource name=w1373, error in (no error)=w1372) -> (VISA resource name out=w1364:refnum<visa-resource-name>, error out=w1363:errorcluster)  [unwired: 1 in]
                          }
                        }
                      }
                    }
                    frame #1 {
                      n282 = VISA Write(VISA resource name=w1389, write buffer="POS? C\n", error in (no error)=w1388) -> (VISA resource name out=w1399:refnum<visa-resource-name>, error out=w1398:errorcluster)  [unwired: 1 out]
                      n283 = VISA Write(VISA resource name=w1385, write buffer="POS? 1\n", error in (no error)=w1384) -> (VISA resource name out=w1401:refnum<visa-resource-name>, error out=w1400:errorcluster)  [unwired: 1 out]
                      n284 = VISA Read(VISA resource name=w1399, byte count=u32 128, error in (no error)=w1398) -> (VISA resource name out=w1387:refnum<visa-resource-name>, read buffer=w1395:string, error out=w1386:errorcluster)  [unwired: 1 out]
                      n285 = VISA Read(VISA resource name=w1401, byte count=u32 128, error in (no error)=w1400) -> (VISA resource name out=w1383:refnum<visa-resource-name>, read buffer=w1390:string, error out=w1382:errorcluster)  [unwired: 1 out]
                      n286 = Fract/Exp String To Number(string=w1395, offset=1) -> (number=w1380:dbl)  [unwired: 2 in, 1 out]
                      n287 = Fract/Exp String To Number(string=w1390, offset=1) -> (number=w1379:dbl)  [unwired: 2 in, 1 out]
                      n288 = Add(x=w1380, y=w1379) -> (x+y=w1378:dbl)
                      n289 = Subtract(x=230.0, y=w1378) -> (x-y=w1376:dbl)
                      n290 = Build Array (concatenate)(w1406, w1376) -> (w1405:dbl[])
                    }
                  }
                }
              }
            }
          }
          n291 = Compound Arithmetic op=OR(w918, "stop") -> (w949:bool)
          n292 = case shown="False" w892 {
            tunnel: w891 -> [w951 w953]
            tunnel: [w950 w952] -> w890
            frame False {
              n293 = Decrement(x=w951) -> (x-1=w950:i32)
            }
            frame True {
              n294 = Increment(x=w953) -> (x+1=w952:i32)
            }
          }
        }
        n295 = Compound Arithmetic op=OR(w838, w837) -> (w839:bool)
      }
      n296 = call-poly <vilib>:"Array To Matrix.vi"("Real 1D Array"=w771) -> ("Real Matrix (Column Vector)"=w770:T2)
      n297 = Index Array(array=w769, index (col)=0 ("disabled index (col)")) -> (element=w767:dbl[])  [unwired: 1 in]
      n298 = Index Array(array=w769, index (col)=1 ("disabled index (col)")) -> (element=w765:dbl[])  [unwired: 1 in]
      n299 = call <vilib>:"create_plot_surface.vi"("z matrix"=w770, "y vector"=w765, "x vector"=w767) -> ("plots out"=→"3D Graph":refnum<class "Base Datatype.lvclass">[])  [unwired: 2 in, 6 out]
    }
    frame #7 {
      n300 = VISA Write(VISA resource name=w1421, write buffer="MOV C 0\n", error in (no error)=w1420) -> (VISA resource name out=w1417:refnum<visa-resource-name>, error out=w1416:errorcluster)  [unwired: 1 out]
      n301 = VISA Write(VISA resource name=w1411, write buffer=":OUTP off\nSYST:ZCH ON\n", error in (no error)=w1410) -> (VISA resource name out=w1408:refnum<visa-resource-name>, error out=w1407:errorcluster)  [unwired: 1 out]
      n302 = VISA Write(VISA resource name=w1424, write buffer="MOV 1 0\nEER?\n", error in (no error)=w1423) -> (VISA resource name out=w1415:refnum<visa-resource-name>, error out=w1414:errorcluster)  [unwired: 1 out]
      n303 = Wait (ms)(milliseconds to wait=u32 200) -> ()  [unwired: 1 out]
    }
    frame #8 {
      n304 = VISA Write(VISA resource name=w1436, write buffer="MOV A 0\nMOV B 0\nERR?\n", error in (no error)=w1435) -> (VISA resource name out=w1432:refnum<visa-resource-name>, error out=w1431:errorcluster)  [unwired: 1 out]
      n305 = Wait (ms)(milliseconds to wait=u32 200) -> ()  [unwired: 1 out]
    }
  }
  n306 = VISA Close(VISA resource name=w14, error in (no error)=w13) -> ()  [unwired: 1 out]
  n307 = VISA Close(VISA resource name=w18, error in (no error)=w17) -> ()  [unwired: 1 out]
  n308 = VISA Close(VISA resource name=w16, error in (no error)=w15) -> ()  [unwired: 1 out]
